vi "AddNode.vi"(8 "error in (no error)":errorcluster, 9 "Node Name":string, 10 "point":cluster{"x":i16, "y":i16}, 11 "FSM in":refnum<class "FSM.Graph.lvclass">) -> (0 "error out":errorcluster, 3 "FSM out":refnum<class "FSM.Graph.lvclass">)   [LabVIEW 2015, in "FSM.Graph.lvclass"]
uses:
  FSM.Graph.lvclass
  FSM.Graph.lvclass/FSM.Graph.ctl
  FSM.Node/Shape.ctl
  FSM.Node/FSM.Node.lvclass/FSM.Node.ctl
  FSM.Node/Write Shape.vi
  FSM.Node/FSM.Node.lvclass
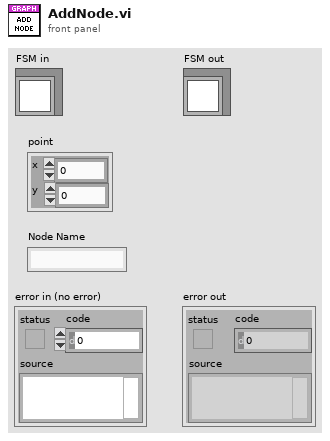
[diagram p1: front panel]
types:
  T1 = typedef "FSM.Node.lvclass/Shape.ctl" = enum16{"Default", "Start", "Action", "End"}
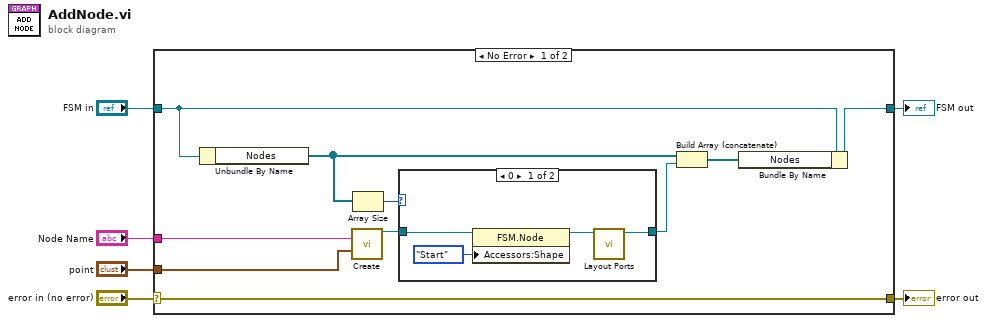
[diagram p0: block diagram]
diagram:
  n1 = case shown="No Error" "error in (no error)" {
    selector: "error in (no error)" -> [w16 w23]
    tunnel: [w16 w23] -> w5
    tunnel: [w13 w22] -> w3
    tunnel: "FSM in" -> [w15 w22]
    tunnel: "Node Name" -> [w7 _]
    tunnel: "point" -> [w14 _]
    frame No Error {
      n2 = Unbundle By Name(w15) -> ("Nodes"=w11:refnum<class "FSM.Node.lvclass">[])
      n3 = call "Create.vi"("Name"=w7, "Center"=w14) -> ("FSM.Node"=w10:refnum<class "FSM.Node.lvclass">)  [unwired: 13 in]
      n4 = Array Size(array=w11) -> (size(s)=w9:i32)
      n5 = case shown="0" w9 {
        tunnel: w10 -> [w20 w21]
        tunnel: [w17 w21] -> w8
        frame 0 {
          n6 = property class="FSM.Node"(reference=w20, "Accessors:Shape"=Shape."Start" ("Shape")) -> (reference out=w18:refnum<class "FSM.Node.lvclass">)  [unwired: 1 in, 1 out]
          n7 = call "Layout Ports.vi"("Node in"=w18) -> ("Node out"=w17:refnum<class "FSM.Node.lvclass">)  [unwired: 9 in, 1 out]
        }
        frame 1, Default {
        }
      }
      n8 = Build Array (concatenate)(w11, w8) -> (w12:refnum<class "FSM.Node.lvclass">[])
      n9 = Bundle By Name(cluster=w15, "Nodes"=w12) -> (w13:refnum<class "FSM.Graph.lvclass">)
    }
    frame Error {
    }
  }
  "error out" <- w5
  "FSM out" <- w3
